vi "Portão de garagem.vi"() -> ()   [LabVIEW 2018]
panel:
  in  "Down Button":bool
  in  "Up Button":bool
  in  "stop":bool
  out "Portão":bool
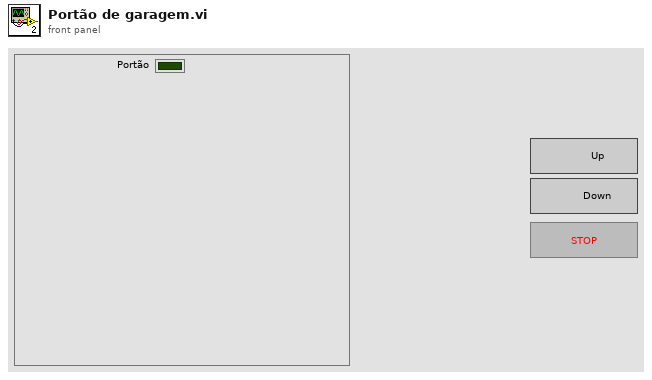
[diagram p1: front panel]
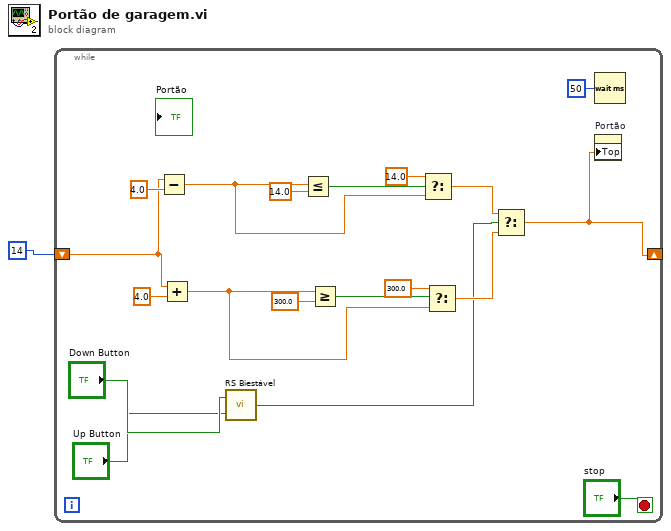
[diagram p0: block diagram]
diagram:
  n1 = while {
    shift-right: [w4] -> _
    shift-left: 14 -> [w16]
    stop <- "stop" stop-if-true
    n2 = Subtract(x=w16, y=4.0) -> (x-y=w11:dbl)
    n3 = Add(x=w16, y=4.0) -> (x+y=w7:dbl)
    n4 = call "RS Biestável.vi"("SET"="Up Button", "RESET"="Down Button") -> ("SAIDA"=w5:bool)
    n5 = Less Or Equal?(x=w11, y=14.0) -> (x <= y?=w13:bool)
    n6 = Greater Or Equal?(x=w7, y=300.0) -> (x >= y?=w9:bool)
    n7 = Select(t=14.0, s=w13, f=w11) -> (s? t:f=w10:dbl)
    n8 = Select(t=300.0, s=w9, f=w7) -> (s? t:f=w6:dbl)
    n9 = Select(t=w10, s=w5, f=w6) -> (s? t:f=w4:dbl)
    n10 = Wait (ms)(milliseconds to wait=u32 50) -> ()  [unwired: 1 out]
    n11 = property on="Portão" class="Bool (strict)"("Top"=w4) -> ()  [unwired: 2 in, 2 out]
  }
